vi "Resize 1D Array.vi"(4 "array size":i32, 5 "input array":dbl[](array[numeric]) format="%.2f") -> (2 "output array":dbl[](array[numeric]) format="%.2f")   [LabVIEW 2020, in "NI_PID_pid.lvlib"]
uses:
  <vilib>/addons/control/pid/NI_PID_pid.lvlib
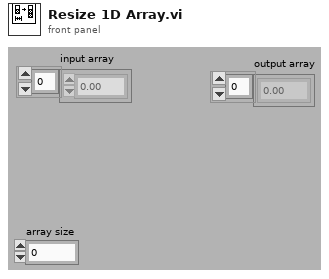
[diagram p1: front panel]
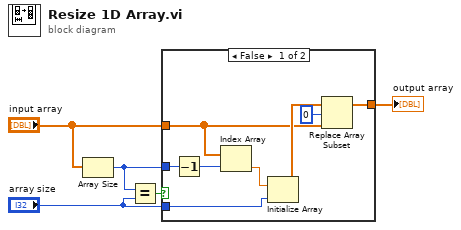
[diagram p0: block diagram]
diagram:
  n1 = Array Size(array="input array") -> (size(s)=w2:i32)
  n2 = Equal?(x=w2, y="array size") -> (x = y?=w5:bool)
  n3 = case shown="False" w5 {
    tunnel: "input array" -> [w7 w14]
    tunnel: [w12 w14] -> w3
    tunnel: "array size" -> [w10 _]
    tunnel: w2 -> [w13 _]
    frame False {
      n4 = Decrement(x=w13) -> (x-1=w11:i32)
      n5 = Index Array(array=w7, index=w11) -> (element=w9:dbl)
      n6 = Initialize Array(w9, w10) -> (w8:dbl[])
      n7 = Replace Array Subset(array=w8, new element=w7, index=0) -> (w12:dbl[])
    }
    frame True {
    }
  }
  "output array" <- w3
